vi "Pet Watchdog.vi"(8 "error in (no error)":errorcluster, 11 "FPGA VI Reference Out":refnum<k20>) -> (0 "error out":errorcluster, 3 "FPGA VI Reference Out 2":refnum<k20>)   [LabVIEW 2015]
uses:
  RT/RT Global References.vi
  <vilib>/Utility/error.llb/Error Cluster From Error Code.vi
  <vilib>/rvi/errors/niLvFpgaAdjustHostInterfaceError.vi
  <vilib>/rvi/interface/nirviReadWriteControl/nirviReadWriteControl.xnode
  NiFpgaLv.dll
  <vilib>/rvi/interface/Simulation/niFpgaSimulationCallBeginRW.vi
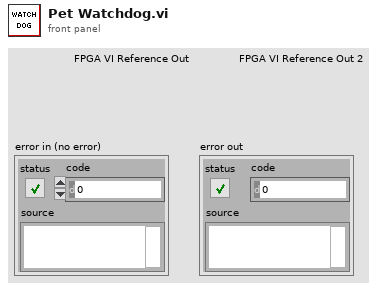
[diagram p1: front panel]
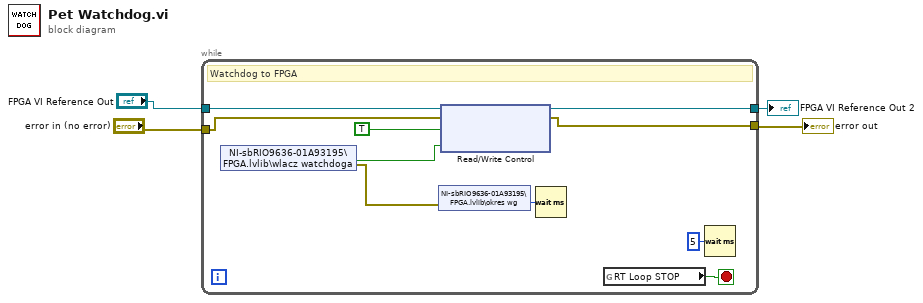
[diagram p0: block diagram]
diagram:
  n1 = while {
    tunnel: "FPGA VI Reference Out" -> [w14]
    tunnel: "error in (no error)" -> [w9]
    tunnel: [w8] -> w1
    tunnel: [w7] -> w3
    stop <- w5 stop-if-true
    # "Watchdog to FPGA"
    n2 = shared-variable "NI-sbRIO9636-01A93195\\FPGA.lvlib\\wlacz watchdoga"() -> (w11:bool, error out=w6:errorcluster)  [unwired: 1 in]
    n3 = shared-variable "NI-sbRIO9636-01A93195\\FPGA.lvlib\\okres wg"(error in=w6) -> (w12:u32)  [unwired: 1 out]
    n4 = xnode "Read/Write Control"("FPGA VI Reference In"=w14, "error in"=w9, "watchdog"=TRUE, "wlacz watchdoga"=w11) -> ("FPGA VI Reference Out"=w8:refnum<k20>, "error out"=w7:errorcluster)
    n5 = Wait (ms)(milliseconds to wait=w12) -> ()  [unwired: 1 out]
    n6 = global read "RT Global References.vi" "RT Loop STOP"() -> (w5:bool)
    n7 = Wait (ms)(milliseconds to wait=u32 5) -> ()  [unwired: 1 out]
  }
  "error out" <- w3
  "FPGA VI Reference Out 2" <- w1
